vi "SLSC Get Module Name from IP Address.vi"(5 "Password":string, 6 "connect timeout":dbl=50.0, 7 "Username":string="admin", 8 "Error In":errorcluster, 9 "Wait for mDSN?":bool, 10 "Slot #":u32=4, 11 "Chassis IP Address":string="192.168.0.14") -> (0 "Error Out":errorcluster, 1 "SLSC Chassis Name":string, 3 "SLSC Module Name":string)   [LabVIEW 2020, in "SLSC CD Engine.lvlib"]
uses:
  SLSC CD Engine.lvlib
  <vilib>/SLSC/SLSC.lvlib
  <resource>/objmgr/slsc.rc
  <vilib>/nisyscfg/nisyscfg.lvlib
  <resource>/objmgr/nisysapi.rc
  <vilib>/nisyscfg/Close (System).vi
  <vilib>/SLSC/Initialize Session without Resources.vi
  <vilib>/SLSC/Initialize Session with Devices.vi
  <vilib>/SLSC/Close Session.vi
panel:
  out "Dev.SlotNum":u32
  out "Module Found?":bool
  out "Host Name":string
  out "Dev.Modules":string[](array[string])
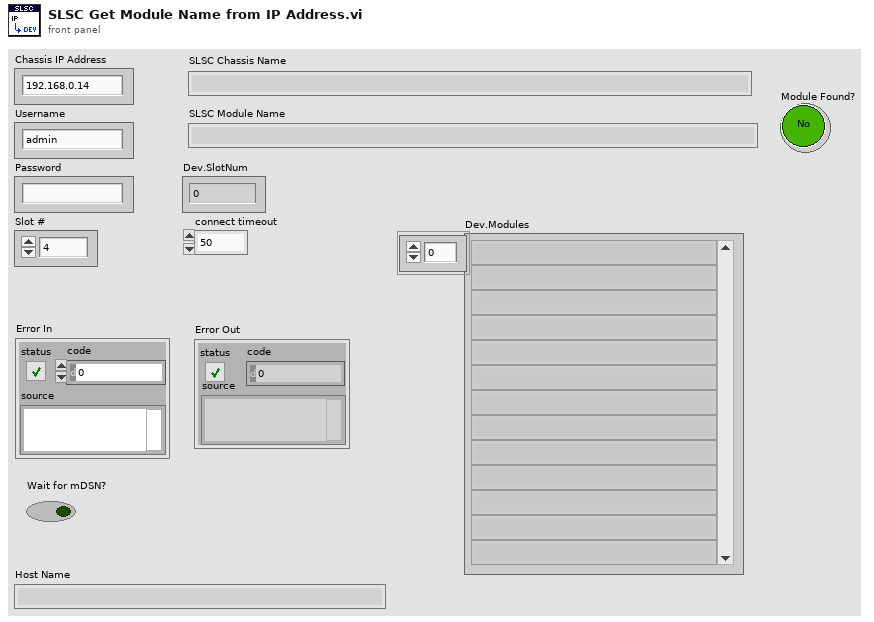
[diagram p1: front panel]
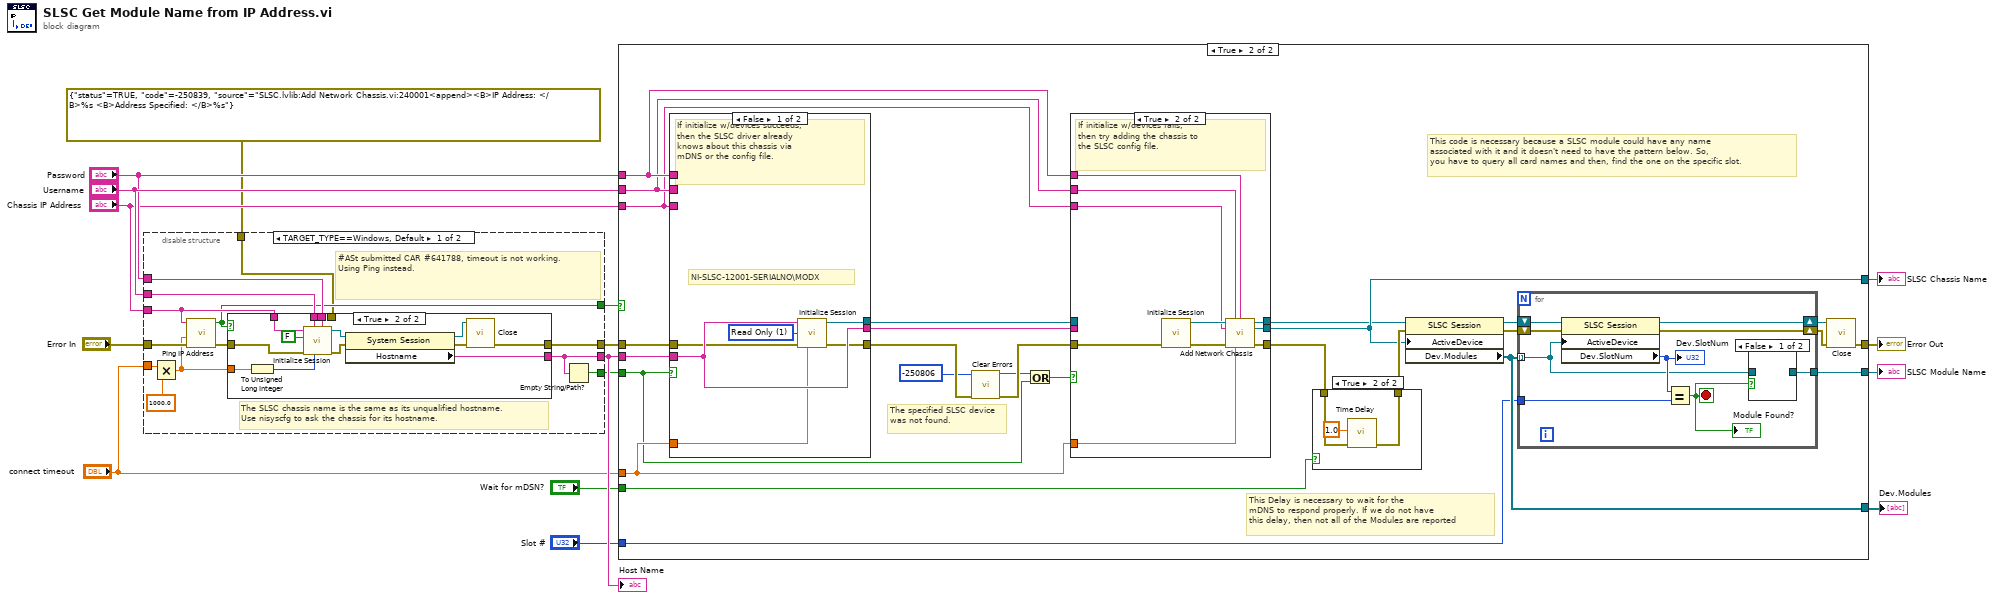
[diagram p0: block diagram]
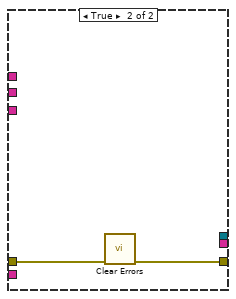
[diagram p5: hidden frame]
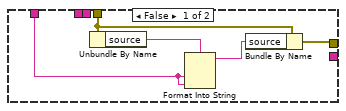
[diagram p7: hidden frame]
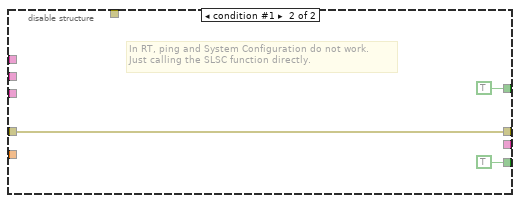
[diagram p8: hidden frame]
diagram:
  n1 = disable-structure shown="TARGET_TYPE==Windows, Default" {
    disable-tunnel: [w29 w49] -> w4
    disable-tunnel: "Username" -> [w28 _]
    disable-tunnel: "Password" -> [w27 _]
    disable-tunnel: [w26 TRUE] -> w5
    disable-tunnel: [w25 _] -> w11
    disable-tunnel: "Chassis IP Address" -> [w24 _]
    disable-tunnel: "Error In" -> [w23 w49]
    disable-tunnel: "connect timeout" -> [w20 _]
    disable-tunnel: [w18 TRUE ("response?")] -> w3
    disable-tunnel: errorcluster {"status"=TRUE, "code"=-250839, "source"="SLSC.lvlib:Add Network Chassis.vi:240001<append><B>IP Address: </B>%s <B>Address Specified: </B>%s"} ("Error Out") -> [w17 _]
    frame condition #0 (active) {
      # "#ASt submitted CAR #641788, timeout is not working.\nUsing Ping instead."
      # "The SLSC chassis name is the same as its unqualified hostname.\nUse nisyscfg to ask the chassis for its hostname."
      n2 = Multiply(x=w20, y=1000.0) -> (x*y=w19:dbl)
      n3 = call "Ping IP Address.vi"("error in"=w23, "timeout (500 ms)"=w19, "host"=w24) -> ("error out"=w22:errorcluster, "response?"=w18:bool)  [unwired: 6 in, 1 out]
      n4 = case shown="True" w18 {
        tunnel: [w32 w43] -> w29
        tunnel: w22 -> [_ w41]
        tunnel: w28 -> [_ w40]
        tunnel: w27 -> [_ w39]
        tunnel: [_ w37] -> w25
        tunnel: w24 -> [w31 w36]
        tunnel: w19 -> [_ w35]
        tunnel: w17 -> [w30 _]
        frame False {
          n5 = Unbundle By Name(w30) -> ("source"=w34:string)
          n6 = Format Into String(format string=w34, w31, w31) -> (resulting string=w33:string)  [unwired: 2 in, 1 out]
          n7 = Bundle By Name(cluster=w30, "source"=w33) -> (w32:errorcluster)
        }
        frame True {
          n8 = To Unsigned Long Integer(number=w35) -> (unsigned 32bit integer=w42:u32)
          n9 = call <vilib>:"Initialize Session.vi"("Password"=w39, "Connect Timeout (4000 ms)"=w42, "User Name"=w40, "error in (no error)"=w41, "Force Property Refresh (T)"=FALSE, "Target (localhost)"=w36) -> ("error out"=w46:errorcluster, "Session out"=w47:refnum<k21>)  [unwired: 4 in]
          n10 = property class="System Session"(reference=w47, error in=w46) -> (reference out=w44:refnum<k21>, error out=w45:errorcluster, "Hostname"=w37:string)
          n11 = call-poly <vilib>:"Close.vi"("error in (no error)"=w45, "Session in"=w44) -> ("error out"=w43:errorcluster)  [unwired: 9 in]
        }
      }
      n12 = Empty String/Path?(string/path=w25) -> (empty?=w26:bool)
    }
    frame condition #1 {
      # "In RT, ping and System Configuration do not work.\nJust calling the SLSC function directly."
    }
  }
  "Host Name" <- w11
  n13 = case shown="True" w3 {
    tunnel: [w51 w78] -> w16
    tunnel: "Username" -> [_ w53]
    tunnel: "Password" -> [_ w54]
    tunnel: [_ w65] -> w13
    tunnel: [_ w77] -> w12
    tunnel: w11 -> [_ w76]
    tunnel: "Chassis IP Address" -> [_ w52]
    tunnel: "connect timeout" -> [_ w60]
    tunnel: [_ w75] -> w7
    tunnel: "Slot #" -> [_ w74]
    tunnel: w5 -> [_ w56]
    tunnel: w4 -> [w51 w68]
    tunnel: "Wait for mDSN?" -> [_ w67]
    frame False {
    }
    frame True {
      # "The specified SLSC device was not found."
      # "This code is necessary because a SLSC module could have any name\nassociated with it and it doesn't need to have the pattern below. So,\nyou have to query all card names and then, find the one on the specific slot."
      # "This Delay is necessary to wait for the \nmDNS to respond properly. If we do not have\nthis delay, then not all of the Modules are reported"
      n14 = case shown="False" w56 {
        tunnel: [w98 w103] -> w63
        tunnel: [w99 _] -> w61
        tunnel: w52 -> [_ _]
        tunnel: w53 -> [_ _]
        tunnel: w54 -> [_ _]
        tunnel: [w100 _] -> w62
        tunnel: w76 -> [w100 _]
        tunnel: w60 -> [w96 _]
        tunnel: w68 -> [w97 w102]
        frame False {
          w101 = 1 items=["None"=0, "Read Only"=1, "Read/Write"=3] ("reservation access (Read/Write)")
          # "NI-SLSC-12001-SERIALNO\\MODX"
          # "If initialize w/devices succeeds,\nthen the SLSC driver already\nknows about this chassis via\nmDNS or the config file."
          n15 = call-poly <vilib>:"Initialize Session.vi"("devices"=w100, "reservation access (Read/Write)"=w101, "error in (no error)"=w97, "connect timeout (60 sec)"=w96) -> ("session out"=w99:refnum<k21>, "error out"=w98:errorcluster)  [unwired: 10 in]
        }
        frame True {
          n16 = call <vilib>:"Clear Errors.vi"("error in (no error)"=w102) -> ("error out"=w103:errorcluster)  [unwired: 5 in, 1 out]
        }
      }
      n17 = call <vilib>:"Clear Errors.vi"("error in (no error)"=w63, "specific error code to clear (0: all)"=-250806) -> ("error out"=w59:errorcluster, "specific error cleared?"=w57:bool)  [unwired: 4 in]
      n18 = Or(x=w57, y=w56) -> (x .or. y?=w55:bool)
      n19 = case shown="True" w55 {
        tunnel: [w81 w84] -> w66
        tunnel: [w79 w85] -> w64
        tunnel: w52 -> [_ w90]
        tunnel: w53 -> [_ w88]
        tunnel: w54 -> [_ w87]
        tunnel: [w80 w86] -> w65
        tunnel: w60 -> [_ w83]
        tunnel: w59 -> [w81 w82]
        tunnel: w62 -> [w80 _]
        tunnel: w61 -> [w79 _]
        frame False {
        }
        frame True {
          # "If initialize w/devices fails,\nthen try adding the chassis to\nthe SLSC config file."
          n20 = call-poly <vilib>:"Initialize Session.vi"("error in (no error)"=w82) -> ("session out"=w91:refnum<k21>, "error out"=w89:errorcluster)  [unwired: 13 in]
          n21 = call <vilib>:"Add Network Chassis.vi"("session in"=w91, "username"=w88, "password"=w87, "chassis IP address/hostname"=w90, "error in (no error)"=w89, "connect timeout (60 sec)"=w83) -> ("session out"=w85:refnum<k21>, "chassis out"=w86:refnum<k21>, "error out"=w84:errorcluster)  [unwired: 7 in]
        }
      }
      n22 = case shown="True" w67 {
        tunnel: w66 -> [w92 w95]
        tunnel: [w92 w94] -> w69
        frame False {
        }
        frame True {
          n23 = call "Time Delay"("error in (no error)"=w95, "Delay Time (s)"=1.0) -> ("error out"=w94:errorcluster)  [unwired: 9 in]
        }
      }
      n24 = property class="SLSC Session"(reference=w64, error in=w69, "ActiveDevice"=w65) -> (reference out=w73:refnum<k21>, error out=w72:errorcluster, "Dev.Modules"=w75:refnum<k21>[])
      n25 = for {
        tunnel: w75 -> [w106] mode=indexing
        tunnel: w74 -> [w112]
        tunnel: [w105] -> w77
        shift-right: [w108] -> w70
        shift-left: w72 -> [w109]
        shift-right: [w107] -> w71
        shift-left: w73 -> [w111]
        stop <- w104 stop-if-true
        n26 = property class="SLSC Session"(reference=w111, error in=w109, "ActiveDevice"=w106) -> (reference out=w107:refnum<k21>, error out=w108:errorcluster, "Dev.SlotNum"=w110:u32)
        "Dev.SlotNum" <- w110
        n27 = Equal?(x=w110, y=w112) -> (x = y?=w104:bool)
        "Module Found?" <- w104
        n28 = case shown="False" w104 {
          tunnel: w106 -> [_ w113]
          tunnel: [_ w113] -> w105
          frame False {
          }
          frame True {
          }
        }
      }
      n29 = call-poly <vilib>:"Close.vi"("session in"=w71, "error in (no error)"=w70) -> ("error out"=w78:errorcluster)  [unwired: 13 in]
    }
  }
  "SLSC Chassis Name" <- w13
  "Error Out" <- w16
  "SLSC Module Name" <- w12
  "Dev.Modules" <- w7
